vi "AprilTagFieldLayout_New2025.vi"() -> (3 "AprilTagFieldLayout":T1={"AprilTagMap"={}, "FieldLength"=0.0, "FieldWidth"=0.0, "OriginPosition "=enum."kBlueAllianceWallRightSide,", "OriginPose3d"={"Translation3d"={"X"=0.0, "Y"=0.0, "Z"=0.0}, "Rotation3d"={"Q_quaternion"={"R"=1.0, "V"=[0.0, 0.0, 0.0]}}}} {"OriginPose3d"."Translation3d"."Z" format="%14.3f"; "OriginPose3d"."Translation3d"."Y" format="%14.3f"; "OriginPose3d"."Translation3d"."X" format="%14.3f"})   [LabVIEW 2019, in "Trajectory_Library.lvlib"]
doc: "Define the FRC 2025 April Tag field layout.\n\nInputs:\n <none>\n\nOutputs:\n -- AprilTagFieldLayout -- AprilTagFieldLayout -- Data cluster containing field definition."
uses:
  TypeDef/AprilTagFieldLayout.ctl
  TypeDef/AprilTag.ctl
  TypeDef/POSE3D.ctl
  TypeDef/TRANSLATION3D.ctl
  TypeDef/ROTATION3D.ctl
  TypeDef/QUATERNION.ctl
  Enum/AprilTagFieldLayoutOrignPosition_ENUM.ctl
  AprilTag_GetAll.vi
  Quaternion_Normalize.vi
  Quaternion_New_Default.vi
  Trajectory_Library.lvlib
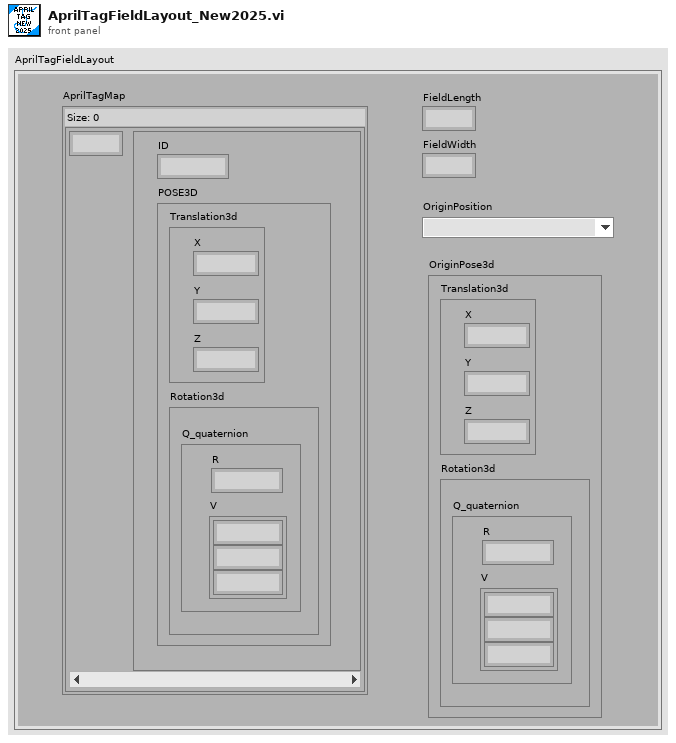
[diagram p1: front panel]
types:
  T1 = typedef "Trajectory_Library.lvlib/AprilTagFieldLayout.ctl" = cluster{"AprilTagMap":map{i32, T2}, "FieldLength":dbl, "FieldWidth":dbl, "OriginPosition ":T7, "OriginPose3d":T3}
  T2 = typedef "Trajectory_Library.lvlib/AprilTag.ctl" = cluster{"ID":i32, "POSE3D":T3}
  T3 = typedef "Trajectory_Library.lvlib/POSE3D.ctl" = cluster{"Translation3d":T4, "Rotation3d":T5}
  T4 = typedef "Trajectory_Library.lvlib/TRANSLATION3D.ctl" = cluster{"X":dbl, "Y":dbl, "Z":dbl}
  T5 = typedef "Trajectory_Library.lvlib/ROTATION3D.ctl" = cluster{"Q_quaternion":T6}
  T6 = typedef "Trajectory_Library.lvlib/QUATERNION.ctl" = cluster{"R":dbl, "V":dbl[]}
  T7 = typedef "Trajectory_Library.lvlib/AprilTagFieldLayoutOrignPosition_ENUM.ctl" = enum16{"kBlueAllianceWallRightSide,", "kRedAllianceWallRightSide,"}
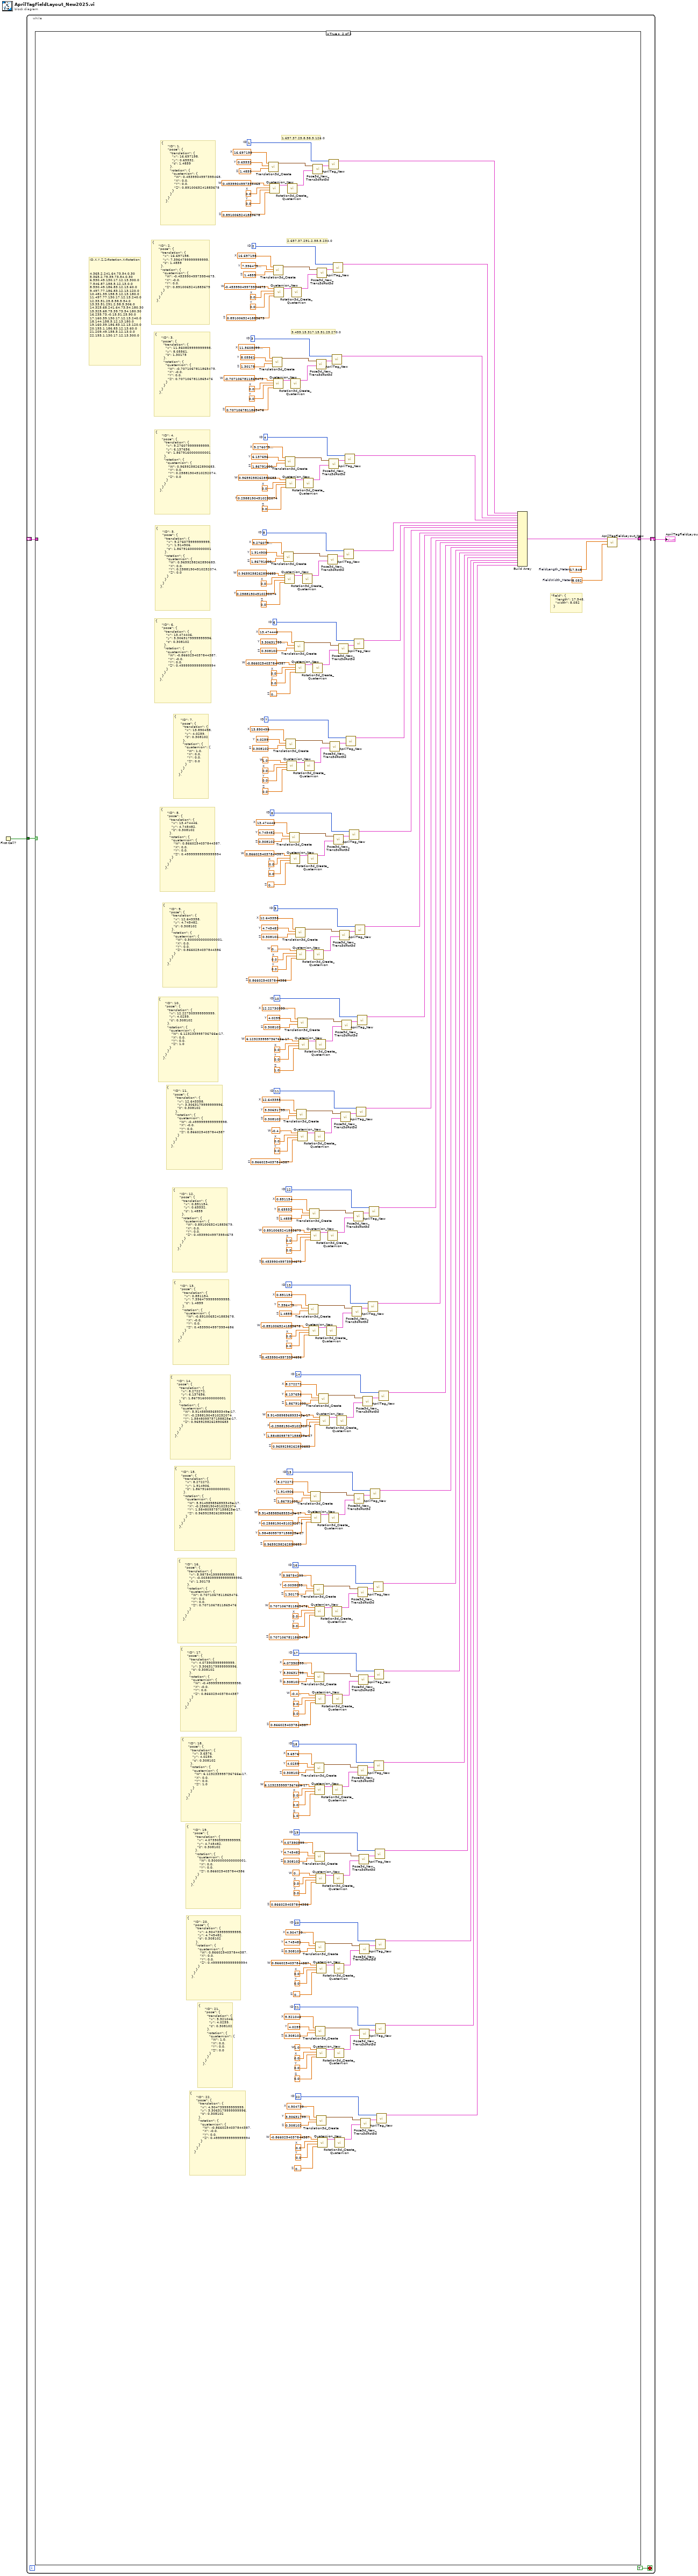
[diagram p0: block diagram]
diagram:
  n1 = First Call?() -> (First Call?: T/F=w1:bool)
  n2 = while {
    shift-right: [w6] -> w2
    shift-left: _ -> [w3]
    tunnel: w1 -> [w4]
    stop <- TRUE stop-if-true
    n3 = case shown="True" w4 {
      tunnel: [w7 w297] -> w6
      tunnel: w3 -> [w7 _]
      frame False {
      }
      frame True {
        w15 = 22  # ID
        w17 = 4.904739999999999  # X
        w18 = 3.3063179999999996  # Y
        w19 = 0.308102  # Z
        w16 = -0.8660254037844387  # W
        w20 = 0.0  # X
        w21 = 0.0  # Y
        w22 = 0.49999999999999994  # Z
        w27 = 21  # ID
        w29 = 5.321046  # X
        w30 = 4.0259  # Y
        w31 = 0.308102  # Z
        w28 = 1.0  # W
        w32 = 0.0  # X
        w33 = 0.0  # Y
        w34 = 0.0  # Z
        w39 = 20  # ID
        w41 = 4.904739999999999  # X
        w42 = 4.745482  # Y
        w43 = 0.308102  # Z
        w40 = 0.8660254037844387  # W
        w44 = 0.0  # X
        w45 = 0.0  # Y
        w46 = 0.49999999999999994  # Z
        w51 = 19  # ID
        w53 = 4.073905999999999  # X
        w54 = 4.745482  # Y
        w55 = 0.308102  # Z
        w52 = 0.5000000000000001  # W
        w56 = 0.0  # X
        w57 = 0.0  # Y
        w58 = 0.8660254037844386  # Z
        w63 = 18  # ID
        w65 = 3.6576  # X
        w66 = 4.0259  # Y
        w67 = 0.308102  # Z
        w64 = 6.123233995736766e-17  # W
        w68 = 0.0  # X
        w69 = 0.0  # Y
        w70 = 1.0  # Z
        w75 = 17  # ID
        w77 = 4.073905999999999  # X
        w78 = 3.3063179999999996  # Y
        w79 = 0.308102  # Z
        w76 = -0.4999999999999998  # W
        w80 = 0.0  # X
        w81 = 0.0  # Y
        w82 = 0.8660254037844387  # Z
        w95 = 16  # ID
        w97 = 5.9875419999999995  # X
        w98 = -0.0038099999999999996  # Y
        w99 = 1.30175  # Z
        w96 = 0.7071067811865476  # W
        w100 = 0.0  # X
        w101 = 0.0  # Y
        w102 = 0.7071067811865476  # Z
        w107 = 15  # ID
        w109 = 8.272272  # X
        w110 = 1.914906  # Y
        w111 = 1.8679160000000001  # Z
        w108 = 5.914589856893349e-17  # W
        w112 = -0.25881904510252074  # X
        w113 = 1.5848095757158825e-17  # Y
        w114 = 0.9659258262890683  # Z
        w119 = 14  # ID
        w121 = 8.272272  # X
        w122 = 6.137656  # Y
        w123 = 1.8679160000000001  # Z
        w120 = 5.914589856893349e-17  # W
        w124 = -0.25881904510252074  # X
        w125 = 1.5848095757158825e-17  # Y
        w126 = 0.9659258262890683  # Z
        w131 = 13  # ID
        w133 = 0.851154  # X
        w134 = 7.3964799999999995  # Y
        w135 = 1.4859  # Z
        w132 = -0.8910065241883678  # W
        w136 = 0.0  # X
        w137 = 0.0  # Y
        w138 = 0.45399049973954686  # Z
        w143 = 12  # ID
        w145 = 0.851154  # X
        w146 = 0.65532  # Y
        w147 = 1.4859  # Z
        w144 = 0.8910065241883679  # W
        w148 = 0.0  # X
        w149 = 0.0  # Y
        w150 = 0.45399049973954675  # Z
        w155 = 11  # ID
        w157 = 12.643358  # X
        w158 = 3.3063179999999996  # Y
        w159 = 0.308102  # Z
        w156 = -0.4999999999999998  # W
        w160 = 0.0  # X
        w161 = 0.0  # Y
        w162 = 0.8660254037844387  # Z
        w167 = 10  # ID
        w169 = 12.227305999999999  # X
        w170 = 4.0259  # Y
        w171 = 0.308102  # Z
        w168 = 6.123233995736766e-17  # W
        w172 = 0.0  # X
        w173 = 0.0  # Y
        w174 = 1.0  # Z
        w179 = 9  # ID
        w181 = 12.643358  # X
        w182 = 4.745482  # Y
        w183 = 0.308102  # Z
        w180 = 0.5000000000000001  # W
        w184 = 0.0  # X
        w185 = 0.0  # Y
        w186 = 0.8660254037844386  # Z
        w200 = 8  # ID
        w202 = 13.474446  # X
        w203 = 4.745482  # Y
        w204 = 0.308102  # Z
        w201 = 0.8660254037844387  # W
        w205 = 0.0  # X
        w206 = 0.0  # Y
        w207 = 0.49999999999999994  # Z
        w212 = 7  # ID
        w214 = 13.890498  # X
        w215 = 4.0259  # Y
        w216 = 0.308102  # Z
        w213 = 1.0  # W
        w217 = 0.0  # X
        w218 = 0.0  # Y
        w219 = 0.0  # Z
        w224 = 6  # ID
        w226 = 13.474446  # X
        w227 = 3.3063179999999996  # Y
        w228 = 0.308102  # Z
        w225 = -0.8660254037844387  # W
        w229 = 0.0  # X
        w230 = 0.0  # Y
        w231 = 0.49999999999999994  # Z
        w236 = 5  # ID
        w238 = 9.276079999999999  # X
        w239 = 1.914906  # Y
        w240 = 1.8679160000000001  # Z
        w237 = 0.9659258262890683  # W
        w241 = 0.0  # X
        w242 = 0.25881904510252074  # Y
        w243 = 0.0  # Z
        w248 = 4  # ID
        w250 = 9.276079999999999  # X
        w251 = 6.137656  # Y
        w252 = 1.8679160000000001  # Z
        w249 = 0.9659258262890683  # W
        w253 = 0.0  # X
        w254 = 0.25881904510252074  # Y
        w255 = 0.0  # Z
        w260 = 3  # ID
        w262 = 11.560809999999998  # X
        w263 = 8.05561  # Y
        w264 = 1.30175  # Z
        w261 = -0.7071067811865475  # W
        w265 = 0.0  # X
        w266 = 0.0  # Y
        w267 = 0.7071067811865476  # Z
        w272 = 2  # ID
        w274 = 16.697198  # X
        w275 = 7.3964799999999995  # Y
        w276 = 1.4859  # Z
        w273 = -0.45399049973954675  # W
        w277 = 0.0  # X
        w278 = 0.0  # Y
        w279 = 0.8910065241883679  # Z
        w284 = 1  # ID
        w286 = 16.697198  # X
        w287 = 0.65532  # Y
        w288 = 1.4859  # Z
        w285 = 0.4539904997395468  # W
        w289 = 0.0  # X
        w290 = 0.0  # Y
        w291 = 0.8910065241883678  # Z
        w295 = 8.052  # FieldWidth_Meters
        w296 = 17.548  # FieldLength_Meters
        # "3,455.15,317.15,51.25,270,0"
        # "2,657.37,291.2,58.5,234,0"
        # "1,657.37,25.8,58.5,126,0"
        # "{\n      \"ID\": 22,\n      \"pose\": {\n        \"translation\": {\n          \"x\": 4.904739999999999,\n          \"y\": 3.3063179999999996,\n          \"z\": 0.308102\n        },\n        \"rotation\": {\n          \"quaternion\": {\n            \"W\": -0.8660254037844387,\n            \"X\": -0.0,\n            \"Y\": 0.0,\n            \"Z\": 0.49999999999999994\n          }\n        }\n      }\n    }"
        # "{\n      \"ID\": 21,\n      \"pose\": {\n        \"translation\": {\n          \"x\": 5.321046,\n          \"y\": 4.0259,\n          \"z\": 0.308102\n        },\n        \"rotation\": {\n          \"quaternion\": {\n            \"W\": 1.0,\n            \"X\": 0.0,\n            \"Y\": 0.0,\n            \"Z\": 0.0\n          }\n        }\n      }\n    },"
        # "{\n      \"ID\": 20,\n      \"pose\": {\n        \"translation\": {\n          \"x\": 4.904739999999999,\n          \"y\": 4.745482,\n          \"z\": 0.308102\n        },\n        \"rotation\": {\n          \"quaternion\": {\n            \"W\": 0.8660254037844387,\n            \"X\": 0.0,\n            \"Y\": 0.0,\n            \"Z\": 0.49999999999999994\n          }\n        }\n      }\n    },"
        # "{\n      \"ID\": 19,\n      \"pose\": {\n        \"translation\": {\n          \"x\": 4.073905999999999,\n          \"y\": 4.745482,\n          \"z\": 0.308102\n        },\n        \"rotation\": {\n          \"quaternion\": {\n            \"W\": 0.5000000000000001,\n            \"X\": 0.0,\n            \"Y\": 0.0,\n            \"Z\": 0.8660254037844386\n          }\n        }\n      }\n    },"
        # "{\n      \"ID\": 18,\n      \"pose\": {\n        \"translation\": {\n          \"x\": 3.6576,\n          \"y\": 4.0259,\n          \"z\": 0.308102\n        },\n        \"rotation\": {\n          \"quaternion\": {\n            \"W\": 6.123233995736766e-17,\n            \"X\": 0.0,\n            \"Y\": 0.0,\n            \"Z\": 1.0\n          }\n        }\n      }\n    },"
        # "{\n      \"ID\": 17,\n      \"pose\": {\n        \"translation\": {\n          \"x\": 4.073905999999999,\n          \"y\": 3.3063179999999996,\n          \"z\": 0.308102\n        },\n        \"rotation\": {\n          \"quaternion\": {\n            \"W\": -0.4999999999999998,\n            \"X\": -0.0,\n            \"Y\": 0.0,\n            \"Z\": 0.8660254037844387\n          }\n        }\n      }\n    },"
        # "\"field\": {\n    \"length\": 17.548,\n    \"width\": 8.052\n  }"
        # "{\n      \"ID\": 16,\n      \"pose\": {\n        \"translation\": {\n          \"x\": 5.9875419999999995,\n          \"y\": -0.0038099999999999996,\n          \"z\": 1.30175\n        },\n        \"rotation\": {\n          \"quaternion\": {\n            \"W\": 0.7071067811865476,\n            \"X\": 0.0,\n            \"Y\": 0.0,\n            \"Z\": 0.7071067811865476\n          }\n        }\n      }\n    },"
        # "{\n      \"ID\": 15,\n      \"pose\": {\n        \"translation\": {\n          \"x\": 8.272272,\n          \"y\": 1.914906,\n          \"z\": 1.8679160000000001\n        },\n        \"rotation\": {\n          \"quaternion\": {\n            \"W\": 5.914589856893349e-17,\n            \"X\": -0.25881904510252074,\n            \"Y\": 1.5848095757158825e-17,\n            \"Z\": 0.9659258262890683\n          }\n        }\n      }\n    },"
        # "{\n      \"ID\": 14,\n      \"pose\": {\n        \"translation\": {\n          \"x\": 8.272272,\n          \"y\": 6.137656,\n          \"z\": 1.8679160000000001\n        },\n        \"rotation\": {\n          \"quaternion\": {\n            \"W\": 5.914589856893349e-17,\n            \"X\": -0.25881904510252074,\n            \"Y\": 1.5848095757158825e-17,\n            \"Z\": 0.9659258262890683\n          }\n        }\n      }\n    },"
        # "{\n      \"ID\": 13,\n      \"pose\": {\n        \"translation\": {\n          \"x\": 0.851154,\n          \"y\": 7.3964799999999995,\n          \"z\": 1.4859\n        },\n        \"rotation\": {\n          \"quaternion\": {\n            \"W\": -0.8910065241883678,\n            \"X\": -0.0,\n            \"Y\": 0.0,\n            \"Z\": 0.45399049973954686\n          }\n        }\n      }\n    },"
        # "{\n      \"ID\": 12,\n      \"pose\": {\n        \"translation\": {\n          \"x\": 0.851154,\n          \"y\": 0.65532,\n          \"z\": 1.4859\n        },\n        \"rotation\": {\n          \"quaternion\": {\n            \"W\": 0.8910065241883679,\n            \"X\": 0.0,\n            \"Y\": 0.0,\n            \"Z\": 0.45399049973954675\n          }\n        }\n      }\n    },"
        # "{\n      \"ID\": 11,\n      \"pose\": {\n        \"translation\": {\n          \"x\": 12.643358,\n          \"y\": 3.3063179999999996,\n          \"z\": 0.308102\n        },\n        \"rotation\": {\n          \"quaternion\": {\n            \"W\": -0.4999999999999998,\n            \"X\": -0.0,\n            \"Y\": 0.0,\n            \"Z\": 0.8660254037844387\n          }\n        }\n      }\n    },"
        # "{\n      \"ID\": 10,\n      \"pose\": {\n        \"translation\": {\n          \"x\": 12.227305999999999,\n          \"y\": 4.0259,\n          \"z\": 0.308102\n        },\n        \"rotation\": {\n          \"quaternion\": {\n            \"W\": 6.123233995736766e-17,\n            \"X\": 0.0,\n            \"Y\": 0.0,\n            \"Z\": 1.0\n          }\n        }\n      }\n    },"
        # "{\n      \"ID\": 9,\n      \"pose\": {\n        \"translation\": {\n          \"x\": 12.643358,\n          \"y\": 4.745482,\n          \"z\": 0.308102\n        },\n        \"rotation\": {\n          \"quaternion\": {\n            \"W\": 0.5000000000000001,\n            \"X\": 0.0,\n            \"Y\": 0.0,\n            \"Z\": 0.8660254037844386\n          }\n        }\n      }\n    },"
        # "{\n      \"ID\": 8,\n      \"pose\": {\n        \"translation\": {\n          \"x\": 13.474446,\n          \"y\": 4.745482,\n          \"z\": 0.308102\n        },\n        \"rotation\": {\n          \"quaternion\": {\n            \"W\": 0.8660254037844387,\n            \"X\": 0.0,\n            \"Y\": 0.0,\n            \"Z\": 0.49999999999999994\n          }\n        }\n      }\n    },"
        # "{\n      \"ID\": 7,\n      \"pose\": {\n        \"translation\": {\n          \"x\": 13.890498,\n          \"y\": 4.0259,\n          \"z\": 0.308102\n        },\n        \"rotation\": {\n          \"quaternion\": {\n            \"W\": 1.0,\n            \"X\": 0.0,\n            \"Y\": 0.0,\n            \"Z\": 0.0\n          }\n        }\n      }\n    },"
        # "{\n      \"ID\": 6,\n      \"pose\": {\n        \"translation\": {\n          \"x\": 13.474446,\n          \"y\": 3.3063179999999996,\n          \"z\": 0.308102\n        },\n        \"rotation\": {\n          \"quaternion\": {\n            \"W\": -0.8660254037844387,\n            \"X\": -0.0,\n            \"Y\": 0.0,\n            \"Z\": 0.49999999999999994\n          }\n        }\n      }\n    },"
        # "{\n      \"ID\": 5,\n      \"pose\": {\n        \"translation\": {\n          \"x\": 9.276079999999999,\n          \"y\": 1.914906,\n          \"z\": 1.8679160000000001\n        },\n        \"rotation\": {\n          \"quaternion\": {\n            \"W\": 0.9659258262890683,\n            \"X\": 0.0,\n            \"Y\": 0.25881904510252074,\n            \"Z\": 0.0\n          }\n        }\n      }\n    },"
        # "{\n      \"ID\": 4,\n      \"pose\": {\n        \"translation\": {\n          \"x\": 9.276079999999999,\n          \"y\": 6.137656,\n          \"z\": 1.8679160000000001\n        },\n        \"rotation\": {\n          \"quaternion\": {\n            \"W\": 0.9659258262890683,\n            \"X\": 0.0,\n            \"Y\": 0.25881904510252074,\n            \"Z\": 0.0\n          }\n        }\n      }\n    },"
        # "{\n      \"ID\": 3,\n      \"pose\": {\n        \"translation\": {\n          \"x\": 11.560809999999998,\n          \"y\": 8.05561,\n          \"z\": 1.30175\n        },\n        \"rotation\": {\n          \"quaternion\": {\n            \"W\": -0.7071067811865475,\n            \"X\": -0.0,\n            \"Y\": 0.0,\n            \"Z\": 0.7071067811865476\n          }\n        }\n      }\n    },"
        # "{\n      \"ID\": 2,\n      \"pose\": {\n        \"translation\": {\n          \"x\": 16.697198,\n          \"y\": 7.3964799999999995,\n          \"z\": 1.4859\n        },\n        \"rotation\": {\n          \"quaternion\": {\n            \"W\": -0.45399049973954675,\n            \"X\": -0.0,\n            \"Y\": 0.0,\n            \"Z\": 0.8910065241883679\n          }\n        }\n      }\n    },"
        # "{\n      \"ID\": 1,\n      \"pose\": {\n        \"translation\": {\n          \"x\": 16.697198,\n          \"y\": 0.65532,\n          \"z\": 1.4859\n        },\n        \"rotation\": {\n          \"quaternion\": {\n            \"W\": 0.4539904997395468,\n            \"X\": 0.0,\n            \"Y\": 0.0,\n            \"Z\": 0.8910065241883678\n          }\n        }\n      }\n    },"
        # "ID,X,Y,Z,Z-Rotation,X-Rotation\n\n\n\n4,365.2,241.64,73.54,0,30\n5,365.2,75.39,73.54,0,30\n6,530.49,130.17,12.13,300,0\n7,546.87,158.5,12.13,0,0\n8,530.49,186.83,12.13,60,0\n9,497.77,186.83,12.13,120,0\n10,481.39,158.5,12.13,180,0\n11,497.77,130.17,12.13,240,0\n12,33.51,25.8,58.5,54,0\n13,33.51,291.2,58.5,306,0\n14,325.68,241.64,73.54,180,30\n15,325.68,75.39,73.54,180,30\n16,235.73,-0.15,51.25,90,0\n17,160.39,130.17,12.13,240,0\n18,144,158.5,12.13,180,0\n19,160.39,186.83,12.13,120,0\n20,193.1,186.83,12.13,60,0\n21,209.49,158.5,12.13,0,0\n22,193.1,130.17,12.13,300,0"
        n4 = call "Translation3d_Create.vi"("Z"=w288, "Y"=w287, "X"=w286) -> ("TRANSLATION3D"=w294:T4)  [unwired: 8 in]
        n5 = call "Quaternion_New.vi"("Z"=w291, "Y"=w290, "X"=w289, "W"=w285) -> ("out Quaternion"=w292:T6)  [unwired: 7 in]
        n6 = call "Translation3d_Create.vi"("Z"=w264, "Y"=w263, "X"=w262) -> ("TRANSLATION3D"=w270:T4)  [unwired: 8 in]
        n7 = call "Translation3d_Create.vi"("Z"=w276, "Y"=w275, "X"=w274) -> ("TRANSLATION3D"=w282:T4)  [unwired: 8 in]
        n8 = call "Quaternion_New.vi"("Z"=w267, "Y"=w266, "X"=w265, "W"=w261) -> ("out Quaternion"=w268:T6)  [unwired: 7 in]
        n9 = call "Quaternion_New.vi"("Z"=w279, "Y"=w278, "X"=w277, "W"=w273) -> ("out Quaternion"=w280:T6)  [unwired: 7 in]
        n10 = call "Translation3d_Create.vi"("Z"=w240, "Y"=w239, "X"=w238) -> ("TRANSLATION3D"=w246:T4)  [unwired: 8 in]
        n11 = call "Quaternion_New.vi"("Z"=w243, "Y"=w242, "X"=w241, "W"=w237) -> ("out Quaternion"=w244:T6)  [unwired: 7 in]
        n12 = call "Translation3d_Create.vi"("Z"=w252, "Y"=w251, "X"=w250) -> ("TRANSLATION3D"=w258:T4)  [unwired: 8 in]
        n13 = call "Quaternion_New.vi"("Z"=w255, "Y"=w254, "X"=w253, "W"=w249) -> ("out Quaternion"=w256:T6)  [unwired: 7 in]
        n14 = call "Translation3d_Create.vi"("Z"=w216, "Y"=w215, "X"=w214) -> ("TRANSLATION3D"=w222:T4)  [unwired: 8 in]
        n15 = call "Quaternion_New.vi"("Z"=w219, "Y"=w218, "X"=w217, "W"=w213) -> ("out Quaternion"=w220:T6)  [unwired: 7 in]
        n16 = call "Rotation3d_Create_Quaternion.vi"("Quaternion"=w292) -> ("Rotation3d"=w293:T5)  [unwired: 10 in]
        n17 = call "Translation3d_Create.vi"("Z"=w204, "Y"=w203, "X"=w202) -> ("TRANSLATION3D"=w210:T4)  [unwired: 8 in]
        n18 = call "Quaternion_New.vi"("Z"=w207, "Y"=w206, "X"=w205, "W"=w201) -> ("out Quaternion"=w208:T6)  [unwired: 7 in]
        n19 = call "Rotation3d_Create_Quaternion.vi"("Quaternion"=w268) -> ("Rotation3d"=w269:T5)  [unwired: 10 in]
        n20 = call "Rotation3d_Create_Quaternion.vi"("Quaternion"=w280) -> ("Rotation3d"=w281:T5)  [unwired: 10 in]
        n21 = call "Translation3d_Create.vi"("Z"=w228, "Y"=w227, "X"=w226) -> ("TRANSLATION3D"=w234:T4)  [unwired: 8 in]
        n22 = call "Quaternion_New.vi"("Z"=w231, "Y"=w230, "X"=w229, "W"=w225) -> ("out Quaternion"=w232:T6)  [unwired: 7 in]
        n23 = call "Translation3d_Create.vi"("Z"=w183, "Y"=w182, "X"=w181) -> ("TRANSLATION3D"=w189:T4)  [unwired: 8 in]
        n24 = call "Quaternion_New.vi"("Z"=w186, "Y"=w185, "X"=w184, "W"=w180) -> ("out Quaternion"=w187:T6)  [unwired: 7 in]
        n25 = call "Translation3d_Create.vi"("Z"=w159, "Y"=w158, "X"=w157) -> ("TRANSLATION3D"=w165:T4)  [unwired: 8 in]
        n26 = call "Translation3d_Create.vi"("Z"=w171, "Y"=w170, "X"=w169) -> ("TRANSLATION3D"=w177:T4)  [unwired: 8 in]
        n27 = call "Quaternion_New.vi"("Z"=w162, "Y"=w161, "X"=w160, "W"=w156) -> ("out Quaternion"=w163:T6)  [unwired: 7 in]
        n28 = call "Quaternion_New.vi"("Z"=w174, "Y"=w173, "X"=w172, "W"=w168) -> ("out Quaternion"=w175:T6)  [unwired: 7 in]
        n29 = call "Rotation3d_Create_Quaternion.vi"("Quaternion"=w244) -> ("Rotation3d"=w245:T5)  [unwired: 10 in]
        n30 = call "Rotation3d_Create_Quaternion.vi"("Quaternion"=w256) -> ("Rotation3d"=w257:T5)  [unwired: 10 in]
        n31 = call "Rotation3d_Create_Quaternion.vi"("Quaternion"=w220) -> ("Rotation3d"=w221:T5)  [unwired: 10 in]
        n32 = call "Rotation3d_Create_Quaternion.vi"("Quaternion"=w208) -> ("Rotation3d"=w209:T5)  [unwired: 10 in]
        n33 = call "Translation3d_Create.vi"("Z"=w135, "Y"=w134, "X"=w133) -> ("TRANSLATION3D"=w141:T4)  [unwired: 8 in]
        n34 = call "Quaternion_New.vi"("Z"=w138, "Y"=w137, "X"=w136, "W"=w132) -> ("out Quaternion"=w139:T6)  [unwired: 7 in]
        n35 = call "Translation3d_Create.vi"("Z"=w147, "Y"=w146, "X"=w145) -> ("TRANSLATION3D"=w153:T4)  [unwired: 8 in]
        n36 = call "Quaternion_New.vi"("Z"=w150, "Y"=w149, "X"=w148, "W"=w144) -> ("out Quaternion"=w151:T6)  [unwired: 7 in]
        n37 = call "Translation3d_Create.vi"("Z"=w111, "Y"=w110, "X"=w109) -> ("TRANSLATION3D"=w117:T4)  [unwired: 8 in]
        n38 = call "Quaternion_New.vi"("Z"=w114, "Y"=w113, "X"=w112, "W"=w108) -> ("out Quaternion"=w115:T6)  [unwired: 7 in]
        n39 = call "Pose3d_New_Trans3dRot3d.vi"("Rotation3d"=w293, "Translation3d"=w294) -> ("outPose3d"=w283:T3)  [unwired: 9 in]
        n40 = call "Rotation3d_Create_Quaternion.vi"("Quaternion"=w232) -> ("Rotation3d"=w233:T5)  [unwired: 10 in]
        n41 = call "Rotation3d_Create_Quaternion.vi"("Quaternion"=w187) -> ("Rotation3d"=w188:T5)  [unwired: 10 in]
        n42 = call "Translation3d_Create.vi"("Z"=w99, "Y"=w98, "X"=w97) -> ("TRANSLATION3D"=w105:T4)  [unwired: 8 in]
        n43 = call "Translation3d_Create.vi"("Z"=w67, "Y"=w66, "X"=w65) -> ("TRANSLATION3D"=w73:T4)  [unwired: 8 in]
        n44 = call "Translation3d_Create.vi"("Z"=w79, "Y"=w78, "X"=w77) -> ("TRANSLATION3D"=w85:T4)  [unwired: 8 in]
        n45 = call "Quaternion_New.vi"("Z"=w102, "Y"=w101, "X"=w100, "W"=w96) -> ("out Quaternion"=w103:T6)  [unwired: 7 in]
        n46 = call "Rotation3d_Create_Quaternion.vi"("Quaternion"=w163) -> ("Rotation3d"=w164:T5)  [unwired: 10 in]
        n47 = call "Quaternion_New.vi"("Z"=w70, "Y"=w69, "X"=w68, "W"=w64) -> ("out Quaternion"=w71:T6)  [unwired: 7 in]
        n48 = call "Translation3d_Create.vi"("Z"=w55, "Y"=w54, "X"=w53) -> ("TRANSLATION3D"=w61:T4)  [unwired: 8 in]
        n49 = call "Quaternion_New.vi"("Z"=w82, "Y"=w81, "X"=w80, "W"=w76) -> ("out Quaternion"=w83:T6)  [unwired: 7 in]
        n50 = call "Translation3d_Create.vi"("Z"=w43, "Y"=w42, "X"=w41) -> ("TRANSLATION3D"=w49:T4)  [unwired: 8 in]
        n51 = call "Translation3d_Create.vi"("Z"=w31, "Y"=w30, "X"=w29) -> ("TRANSLATION3D"=w37:T4)  [unwired: 8 in]
        n52 = call "Rotation3d_Create_Quaternion.vi"("Quaternion"=w175) -> ("Rotation3d"=w176:T5)  [unwired: 10 in]
        n53 = call "Quaternion_New.vi"("Z"=w58, "Y"=w57, "X"=w56, "W"=w52) -> ("out Quaternion"=w59:T6)  [unwired: 7 in]
        n54 = call "Pose3d_New_Trans3dRot3d.vi"("Rotation3d"=w269, "Translation3d"=w270) -> ("outPose3d"=w259:T3)  [unwired: 9 in]
        n55 = call "Quaternion_New.vi"("Z"=w46, "Y"=w45, "X"=w44, "W"=w40) -> ("out Quaternion"=w47:T6)  [unwired: 7 in]
        n56 = call "Quaternion_New.vi"("Z"=w34, "Y"=w33, "X"=w32, "W"=w28) -> ("out Quaternion"=w35:T6)  [unwired: 7 in]
        n57 = call "Translation3d_Create.vi"("Z"=w19, "Y"=w18, "X"=w17) -> ("TRANSLATION3D"=w25:T4)  [unwired: 8 in]
        n58 = call "Pose3d_New_Trans3dRot3d.vi"("Rotation3d"=w281, "Translation3d"=w282) -> ("outPose3d"=w271:T3)  [unwired: 9 in]
        n59 = call "Quaternion_New.vi"("Z"=w22, "Y"=w21, "X"=w20, "W"=w16) -> ("out Quaternion"=w23:T6)  [unwired: 7 in]
        n60 = call "Translation3d_Create.vi"("Z"=w123, "Y"=w122, "X"=w121) -> ("TRANSLATION3D"=w129:T4)  [unwired: 8 in]
        n61 = call "Quaternion_New.vi"("Z"=w126, "Y"=w125, "X"=w124, "W"=w120) -> ("out Quaternion"=w127:T6)  [unwired: 7 in]
        n62 = call "Rotation3d_Create_Quaternion.vi"("Quaternion"=w139) -> ("Rotation3d"=w140:T5)  [unwired: 10 in]
        n63 = call "Pose3d_New_Trans3dRot3d.vi"("Rotation3d"=w245, "Translation3d"=w246) -> ("outPose3d"=w235:T3)  [unwired: 9 in]
        n64 = call "Rotation3d_Create_Quaternion.vi"("Quaternion"=w151) -> ("Rotation3d"=w152:T5)  [unwired: 10 in]
        n65 = call "AprilTag_New.vi"("POSE3D"=w283, "ID"=w284) -> ("AprilTag"=w197:T2)  [unwired: 9 in]
        n66 = call "Rotation3d_Create_Quaternion.vi"("Quaternion"=w115) -> ("Rotation3d"=w116:T5)  [unwired: 10 in]
        n67 = call "Pose3d_New_Trans3dRot3d.vi"("Rotation3d"=w257, "Translation3d"=w258) -> ("outPose3d"=w247:T3)  [unwired: 9 in]
        n68 = call "Pose3d_New_Trans3dRot3d.vi"("Rotation3d"=w221, "Translation3d"=w222) -> ("outPose3d"=w211:T3)  [unwired: 9 in]
        n69 = call "AprilTag_New.vi"("POSE3D"=w259, "ID"=w260) -> ("AprilTag"=w195:T2)  [unwired: 9 in]
        n70 = call "Rotation3d_Create_Quaternion.vi"("Quaternion"=w103) -> ("Rotation3d"=w104:T5)  [unwired: 10 in]
        n71 = call "Rotation3d_Create_Quaternion.vi"("Quaternion"=w71) -> ("Rotation3d"=w72:T5)  [unwired: 10 in]
        n72 = call "Rotation3d_Create_Quaternion.vi"("Quaternion"=w83) -> ("Rotation3d"=w84:T5)  [unwired: 10 in]
        n73 = call "AprilTag_New.vi"("POSE3D"=w271, "ID"=w272) -> ("AprilTag"=w196:T2)  [unwired: 9 in]
        n74 = call "Pose3d_New_Trans3dRot3d.vi"("Rotation3d"=w209, "Translation3d"=w210) -> ("outPose3d"=w199:T3)  [unwired: 9 in]
        n75 = call "Rotation3d_Create_Quaternion.vi"("Quaternion"=w59) -> ("Rotation3d"=w60:T5)  [unwired: 10 in]
        n76 = call "Rotation3d_Create_Quaternion.vi"("Quaternion"=w47) -> ("Rotation3d"=w48:T5)  [unwired: 10 in]
        n77 = call "Rotation3d_Create_Quaternion.vi"("Quaternion"=w35) -> ("Rotation3d"=w36:T5)  [unwired: 10 in]
        n78 = call "Rotation3d_Create_Quaternion.vi"("Quaternion"=w23) -> ("Rotation3d"=w24:T5)  [unwired: 10 in]
        n79 = call "Rotation3d_Create_Quaternion.vi"("Quaternion"=w127) -> ("Rotation3d"=w128:T5)  [unwired: 10 in]
        n80 = call "Pose3d_New_Trans3dRot3d.vi"("Rotation3d"=w233, "Translation3d"=w234) -> ("outPose3d"=w223:T3)  [unwired: 9 in]
        n81 = call "Pose3d_New_Trans3dRot3d.vi"("Rotation3d"=w188, "Translation3d"=w189) -> ("outPose3d"=w178:T3)  [unwired: 9 in]
        n82 = call "Pose3d_New_Trans3dRot3d.vi"("Rotation3d"=w164, "Translation3d"=w165) -> ("outPose3d"=w154:T3)  [unwired: 9 in]
        n83 = call "Pose3d_New_Trans3dRot3d.vi"("Rotation3d"=w176, "Translation3d"=w177) -> ("outPose3d"=w166:T3)  [unwired: 9 in]
        n84 = call "AprilTag_New.vi"("POSE3D"=w235, "ID"=w236) -> ("AprilTag"=w193:T2)  [unwired: 9 in]
        n85 = call "AprilTag_New.vi"("POSE3D"=w247, "ID"=w248) -> ("AprilTag"=w194:T2)  [unwired: 9 in]
        n86 = call "AprilTag_New.vi"("POSE3D"=w211, "ID"=w212) -> ("AprilTag"=w191:T2)  [unwired: 9 in]
        n87 = call "AprilTag_New.vi"("POSE3D"=w199, "ID"=w200) -> ("AprilTag"=w190:T2)  [unwired: 9 in]
        n88 = call "Pose3d_New_Trans3dRot3d.vi"("Rotation3d"=w140, "Translation3d"=w141) -> ("outPose3d"=w130:T3)  [unwired: 9 in]
        n89 = call "Pose3d_New_Trans3dRot3d.vi"("Rotation3d"=w152, "Translation3d"=w153) -> ("outPose3d"=w142:T3)  [unwired: 9 in]
        n90 = call "AprilTag_New.vi"("POSE3D"=w223, "ID"=w224) -> ("AprilTag"=w192:T2)  [unwired: 9 in]
        n91 = call "Pose3d_New_Trans3dRot3d.vi"("Rotation3d"=w116, "Translation3d"=w117) -> ("outPose3d"=w106:T3)  [unwired: 9 in]
        n92 = call "AprilTag_New.vi"("POSE3D"=w178, "ID"=w179) -> ("AprilTag"=w93:T2)  [unwired: 9 in]
        n93 = call "AprilTag_New.vi"("POSE3D"=w154, "ID"=w155) -> ("AprilTag"=w91:T2)  [unwired: 9 in]
        n94 = call "AprilTag_New.vi"("POSE3D"=w166, "ID"=w167) -> ("AprilTag"=w92:T2)  [unwired: 9 in]
        n95 = call "Pose3d_New_Trans3dRot3d.vi"("Rotation3d"=w104, "Translation3d"=w105) -> ("outPose3d"=w94:T3)  [unwired: 9 in]
        n96 = call "Pose3d_New_Trans3dRot3d.vi"("Rotation3d"=w72, "Translation3d"=w73) -> ("outPose3d"=w62:T3)  [unwired: 9 in]
        n97 = call "Pose3d_New_Trans3dRot3d.vi"("Rotation3d"=w84, "Translation3d"=w85) -> ("outPose3d"=w74:T3)  [unwired: 9 in]
        n98 = call "Pose3d_New_Trans3dRot3d.vi"("Rotation3d"=w60, "Translation3d"=w61) -> ("outPose3d"=w50:T3)  [unwired: 9 in]
        n99 = call "Pose3d_New_Trans3dRot3d.vi"("Rotation3d"=w48, "Translation3d"=w49) -> ("outPose3d"=w38:T3)  [unwired: 9 in]
        n100 = call "Pose3d_New_Trans3dRot3d.vi"("Rotation3d"=w36, "Translation3d"=w37) -> ("outPose3d"=w26:T3)  [unwired: 9 in]
        n101 = call "Pose3d_New_Trans3dRot3d.vi"("Rotation3d"=w24, "Translation3d"=w25) -> ("outPose3d"=w14:T3)  [unwired: 9 in]
        n102 = call "Pose3d_New_Trans3dRot3d.vi"("Rotation3d"=w128, "Translation3d"=w129) -> ("outPose3d"=w118:T3)  [unwired: 9 in]
        n103 = call "AprilTag_New.vi"("POSE3D"=w130, "ID"=w131) -> ("AprilTag"=w89:T2)  [unwired: 9 in]
        n104 = call "AprilTag_New.vi"("POSE3D"=w142, "ID"=w143) -> ("AprilTag"=w90:T2)  [unwired: 9 in]
        n105 = call "AprilTag_New.vi"("POSE3D"=w106, "ID"=w107) -> ("AprilTag"=w87:T2)  [unwired: 9 in]
        n106 = call "AprilTag_New.vi"("POSE3D"=w94, "ID"=w95) -> ("AprilTag"=w86:T2)  [unwired: 9 in]
        n107 = call "AprilTag_New.vi"("POSE3D"=w62, "ID"=w63) -> ("AprilTag"=w12:T2)  [unwired: 9 in]
        n108 = call "AprilTag_New.vi"("POSE3D"=w74, "ID"=w75) -> ("AprilTag"=w13:T2)  [unwired: 9 in]
        n109 = call "AprilTag_New.vi"("POSE3D"=w50, "ID"=w51) -> ("AprilTag"=w11:T2)  [unwired: 9 in]
        n110 = call "AprilTag_New.vi"("POSE3D"=w38, "ID"=w39) -> ("AprilTag"=w10:T2)  [unwired: 9 in]
        n111 = call "AprilTag_New.vi"("POSE3D"=w26, "ID"=w27) -> ("AprilTag"=w9:T2)  [unwired: 9 in]
        n112 = call "AprilTag_New.vi"("POSE3D"=w14, "ID"=w15) -> ("AprilTag"=w8:T2)  [unwired: 9 in]
        n113 = call "AprilTag_New.vi"("POSE3D"=w118, "ID"=w119) -> ("AprilTag"=w88:T2)  [unwired: 9 in]
        n114 = Build Array(w197, w196, w195, w194, w193, w192, w191, w190, w93, w92, w91, w90, w89, w88, w87, w86, w13, w12, w11, w10, w9, w8) -> (w198:T2[])
        n115 = call "AprilTagFieldLayout_New.vi"("FieldWidth_Meters"=w295, "FieldLength_Meters"=w296, "AprilTags"=w198) -> ("AprilTagFieldLayout"=w297:T1)  [unwired: 8 in]
      }
    }
  }
  "AprilTagFieldLayout" <- w2
